vi "SIM Adams Change Order.vi"(4 "Adams data":T1, 5 "Current Order":i32, 6 "proposed new order":i32, 7 "Step Accepted?":bool) -> (0 "Adams data out":T1)   [LabVIEW 2014]
uses:
  SIM Adams data.ctl
  SIM Adams stages.ctl
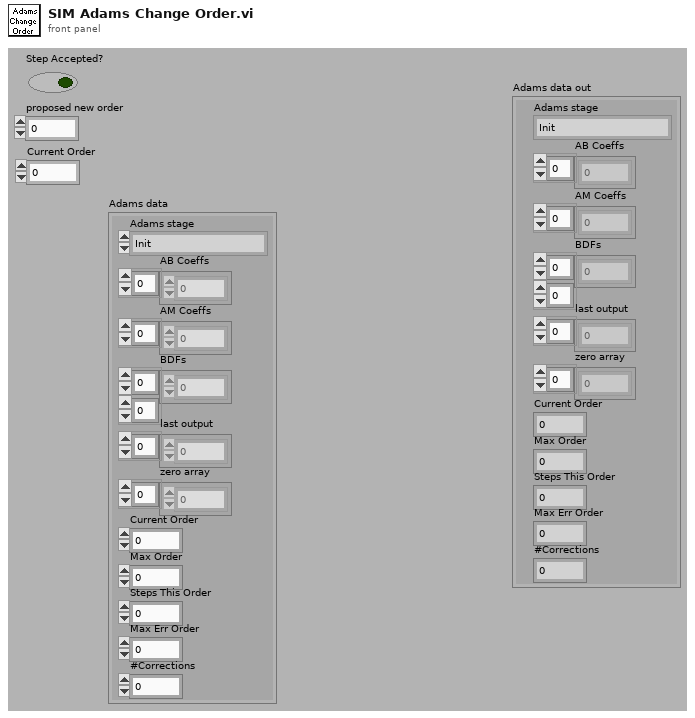
[diagram p1: front panel]
types:
  T1 = typedef "SIM Adams data.ctl" = cluster{"Adams stage":T2, "AB Coeffs":dbl[], "AM Coeffs":dbl[], "BDFs":dbl[][], "last output":dbl[], "zero array":dbl[], "Current Order":i32, "Max Order":i32, "Steps This Order":i32, "Max Err Order":i32, "#Corrections":i32}
  T2 = typedef "SIM Adams stages.ctl" = enum16{"Init", "Predict", "Correct", "Eval Error", "Choose StepSize", "Reset BDFs"}
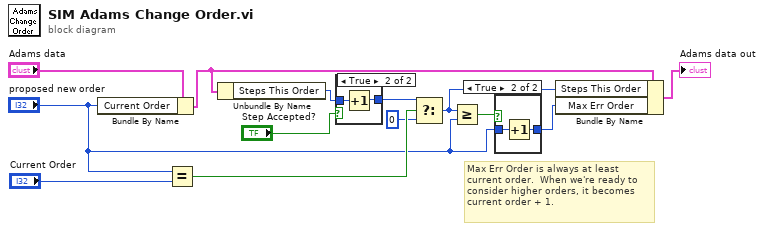
[diagram p0: block diagram]
diagram:
  # "Max Err Order is always at least\ncurrent order.  When we're ready to\nconsider higher orders, it becomes\ncurrent order + 1."
  n1 = Bundle By Name(cluster="Adams data", "Current Order"="proposed new order") -> (w11:T1)
  n2 = Equal?(x="proposed new order", y="Current Order") -> (x = y?=w13:bool)
  n3 = Unbundle By Name(w11) -> ("Steps This Order"=w8:i32)
  n4 = case shown="True" "Step Accepted?" {
    tunnel: w8 -> [w14 w16]
    tunnel: [w14 w15] -> w2
    frame False {
    }
    frame True {
      n5 = Increment(x=w16) -> (x+1=w15:i32)
    }
  }
  n6 = Select(t=w2, s=w13, f=0) -> (s? t:f=w7:i32)
  n7 = Greater Or Equal?(x=w7, y="proposed new order") -> (x >= y?=w5:bool)
  n8 = case shown="True" w5 {
    tunnel: "proposed new order" -> [w17 w19]
    tunnel: [w17 w18] -> w4
    frame False {
    }
    frame True {
      n9 = Increment(x=w19) -> (x+1=w18:i32)
    }
  }
  n10 = Bundle By Name(cluster=w11, "Steps This Order"=w7, "Max Err Order"=w4) -> (→"Adams data out":T1)
